vi "Timestamp to GPS Time.vi"(11 "Timestamp (now)":timestamp) -> (2 "Fractional Second":dbl, 3 "GPS Time (s)":i64)   [LabVIEW 2018]
uses:
  <vilib>/LabVIEW Open Source Project/Epoch Date & Time/epoch.GPS/Epoch.GPS.lvclass
  C:/Program Files (x86)/National Instruments/LabVIEW 2018/vi.lib/LabVIEW Open Source Project/Epoch Date & Time/epoch/Epoch.lvclass
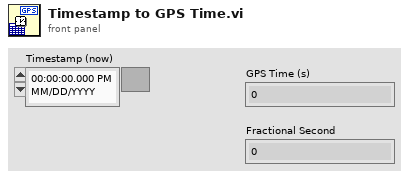
[diagram p1: front panel]
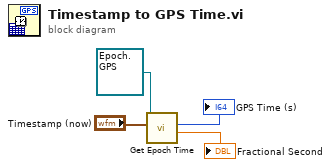
[diagram p0: block diagram]
diagram:
  n1 = call <vilib>:"Get Epoch Time.vi"("Timestamp (now)"="Timestamp (now)", "Epoch (Local)"=refnum<class "Epoch.GPS.lvclass"> refnum ("Epoch.GPS.lvclass")) -> ("Fractional Second"=→"Fractional Second":dbl, "Epoch Time (s)"=→"GPS Time (s)":i64)  [unwired: 7 in, 1 out]
